vi "Show Panel.vi"(8 "error in (no error)":errorcluster, 10 "Panel":refnum<class "Panel.lvclass">, 11 "PanelManager in":refnum<class "PanelManager.lvclass">) -> (0 "error out":errorcluster, 3 "PanelManager out":refnum<class "PanelManager.lvclass">)   [LabVIEW 2018, in "OOPanel.lvlib" / "PanelManager.lvclass"]
uses:
  PanelManager.lvclass
  Panel/Panel.lvclass
  Panel/State.ctl
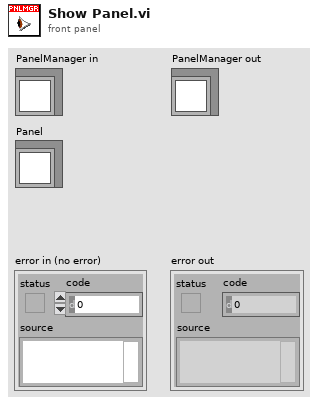
[diagram p1: front panel]
types:
  T1 = typedef "OOPanel.lvlib/Panel.lvclass/State.ctl" = enum16{"Idle", "Hidden", "Visible", "Subpanel"}
  T2 = enum32{"Invalid", "Standard", "Closed", "Hidden", "Minimized", "Maximized"}
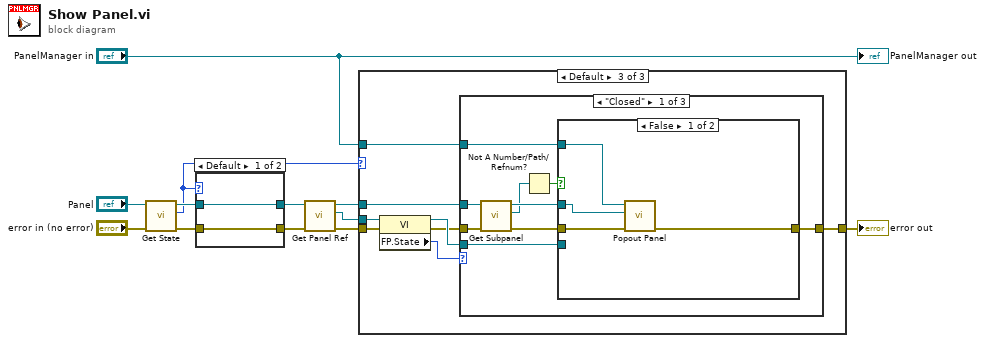
[diagram p0: block diagram]
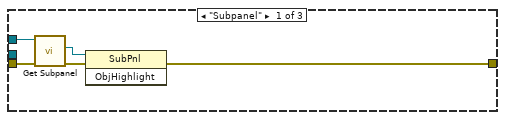
[diagram p2: hidden frame]
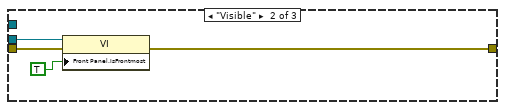
[diagram p3: hidden frame]
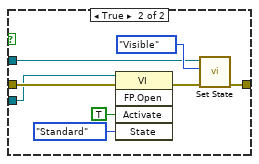
[diagram p4: hidden frame]
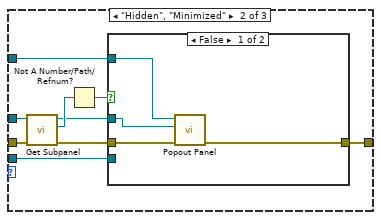
[diagram p5: hidden frame]
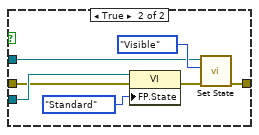
[diagram p6: hidden frame]
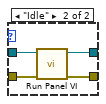
[diagram p8: hidden frame]
diagram:
  n1 = call "Get State.vi"("error in (no error)"="error in (no error)", "Panel in"="Panel") -> ("error out"=w6:errorcluster, "State"=w8:T1, "Panel out"=w9:refnum<class "Panel.lvclass">)  [unwired: 7 in]
  n2 = case shown="Default" w8 {
    tunnel: w9 -> [w14 w18]
    tunnel: [w14 w16] -> w7
    tunnel: w6 -> [w13 w17]
    tunnel: [w13 w15] -> w5
    frame Default {
    }
    frame "Idle" {
      n3 = call "Run Panel VI.vi"("error in (no error)"=w17, "Panel in"=w18) -> ("error out"=w15:errorcluster, "Panel out"=w16:refnum<class "Panel.lvclass">)  [unwired: 8 in]
    }
  }
  n4 = call "Get Panel Ref.vi"("error in (no error)"=w5, "Panel in"=w7) -> ("error out"=w2:errorcluster, "Panel Ref"=w4:refnum<vi>, "Panel out"=w3:refnum<class "Panel.lvclass">)  [unwired: 7 in]
  n5 = case shown="Default" w8 {
    tunnel: [w19 w26 w32] -> w12
    tunnel: w3 -> [w22 _ w30]
    tunnel: w2 -> [w23 w25 w29]
    tunnel: w4 -> [_ w24 w31]
    tunnel: "PanelManager in" -> [_ _ w28]
    frame "Subpanel" {
      n6 = call "Get Subpanel.vi"("error in (no error)"=w23, "Panel in"=w22) -> ("error out"=w20:errorcluster, "Subpanel"=w21:refnum<vi>)  [unwired: 7 in, 1 out]
      n7 = invoke class="SubPnl" method="ObjHighlight"(reference=w21, error in=w20) -> (error out=w19:errorcluster)  [unwired: 1 in, 2 out]
    }
    frame "Visible" {
      n8 = property class="VI"(reference=w24, error in=w25, "Front Panel.IsFrontmost"=TRUE ("Front Panel Window:Is Frontmost")) -> (error out=w26:errorcluster)  [unwired: 1 out]
    }
    frame Default {
      n9 = property class="VI"(reference=w31, error in=w29) -> (reference out=w35:refnum<vi>, error out=w33:errorcluster, "FP.State"=w34:T2)
      n10 = case shown="\"Closed\"" w34 {
        tunnel: w30 -> [w39 w63 _]
        tunnel: w35 -> [w41 w65 _]
        tunnel: w33 -> [w38 w62 w77]
        tunnel: [w36 w64 w77] -> w32
        tunnel: w28 -> [w40 w57 _]
        frame "Closed" {
          n11 = call "Get Subpanel.vi"("error in (no error)"=w38, "Panel in"=w39) -> ("error out"=w42:errorcluster, "Subpanel"=w37:refnum<vi>, "Panel out"=w43:refnum<class "Panel.lvclass">)  [unwired: 7 in]
          n12 = Not A Number/Path/Refnum?(number/path/refnum=w37) -> (NaN/Path/Refnum?=w44:bool)
          n13 = case shown="False" w44 {
            tunnel: w41 -> [_ w51]
            tunnel: [w45 w49] -> w36
            tunnel: w43 -> [w47 w50]
            tunnel: w42 -> [w48 w52]
            tunnel: w40 -> [w46 _]
            frame False {
              n14 = call "Popout Panel.vi"("error in (no error)"=w48, "Panel"=w47, "PanelManager in"=w46) -> ("error out"=w45:errorcluster)  [unwired: 7 in, 1 out]
            }
            frame True {
              n15 = invoke class="VI" method="FP.Open"(reference=w51, error in=w52, "Activate"=TRUE ("Activate?"), "State"=T2."Standard") -> (error out=w56:errorcluster)  [unwired: 1 in, 4 out]
              n16 = call "Set State.vi"("error in (no error)"=w56, "State"=State."Visible", "Panel in"=w50) -> ("error out"=w49:errorcluster)  [unwired: 7 in, 1 out]
            }
          }
        }
        frame "Hidden", "Minimized" {
          n17 = call "Get Subpanel.vi"("error in (no error)"=w62, "Panel in"=w63) -> ("error out"=w58:errorcluster, "Subpanel"=w61:refnum<vi>, "Panel out"=w59:refnum<class "Panel.lvclass">)  [unwired: 7 in]
          n18 = Not A Number/Path/Refnum?(number/path/refnum=w61) -> (NaN/Path/Refnum?=w60:bool)
          n19 = case shown="False" w60 {
            tunnel: w65 -> [_ w75]
            tunnel: [w66 w72] -> w64
            tunnel: w59 -> [w68 w71]
            tunnel: w58 -> [w69 w70]
            tunnel: w57 -> [w67 _]
            frame False {
              n20 = call "Popout Panel.vi"("error in (no error)"=w69, "Panel"=w68, "PanelManager in"=w67) -> ("error out"=w66:errorcluster)  [unwired: 7 in, 1 out]
            }
            frame True {
              n21 = property class="VI"(reference=w75, error in=w70, "FP.State"=T2."Standard" ("Front Panel Window:State")) -> (error out=w73:errorcluster)  [unwired: 1 out]
              n22 = call "Set State.vi"("error in (no error)"=w73, "State"=State."Visible", "Panel in"=w71) -> ("error out"=w72:errorcluster)  [unwired: 7 in, 1 out]
            }
          }
        }
        frame Default {
        }
      }
    }
  }
  "error out" <- w12
  "PanelManager out" <- "PanelManager in"
